vi "Filtering_and_Frequency_Domain.vi"() -> ()   [LabVIEW 2016]
uses:
  <vilib>/Analysis/2dsp.llb/Real FFT.vi
  <vilib>/Analysis/3filter.llb/Butterworth Filter (DBL).vi
  <vilib>/Analysis/NI_AALBase.lvlib
  <vilib>/Analysis/NI_AALPro.lvlib
panel:
  in  "Apply Filter?":bool=TRUE
  in  "Filter Type":T1(ring)
  in  "Low Cutoff Frequency (Hz)":i32=20
  in  "High Cutoff Frequency (Hz)":i32=45
  out "Frequency Domain Signal":cluster{i32, dbl, dbl[]}(graph)={0, 1.0, []}
  in  "Sample Rate (Hz)":dbl=200.0
  out "Time Domain Signal":cluster{i32, dbl, "sine wave":dbl[]}[](graph)
  in  "Frequency (Hz)":dbl=10.0
  in  "Signal Type":enum16{"Impulse", "Sine wave", "Square wave"}(ring)
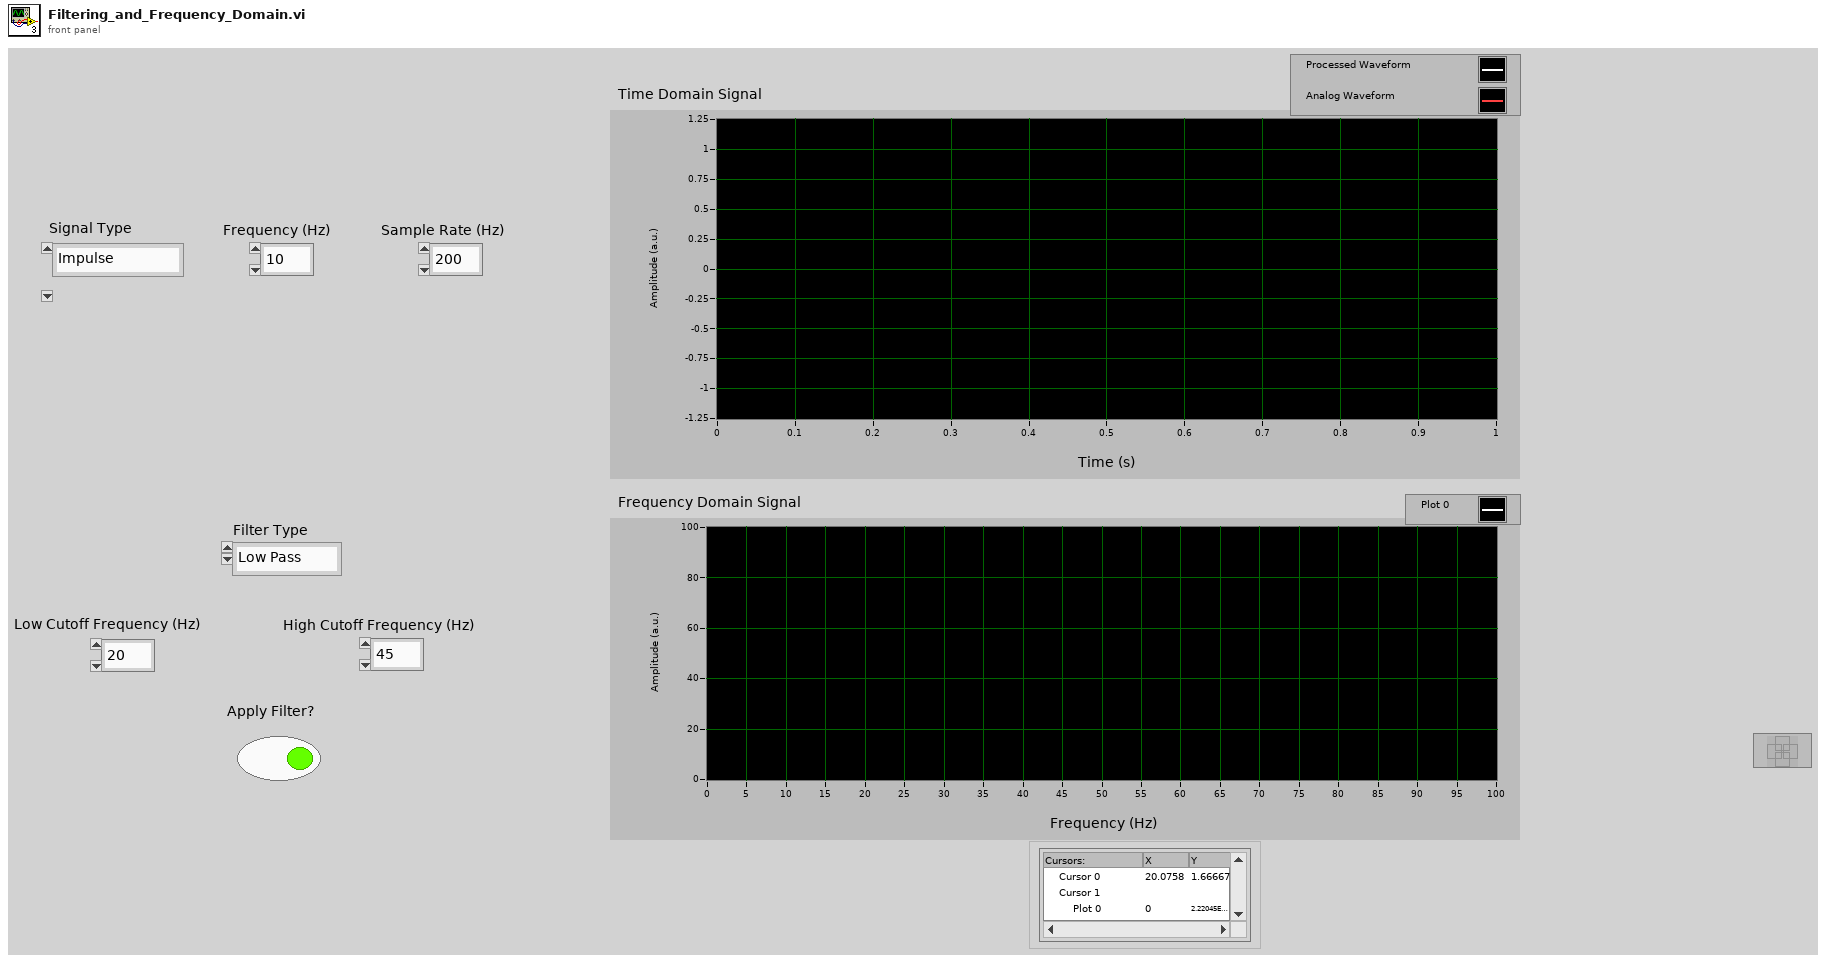
[diagram p1: front panel]
types:
  T1 = enum16{"Low Pass", "High Pass", "Band Pass", "Band Stop"}
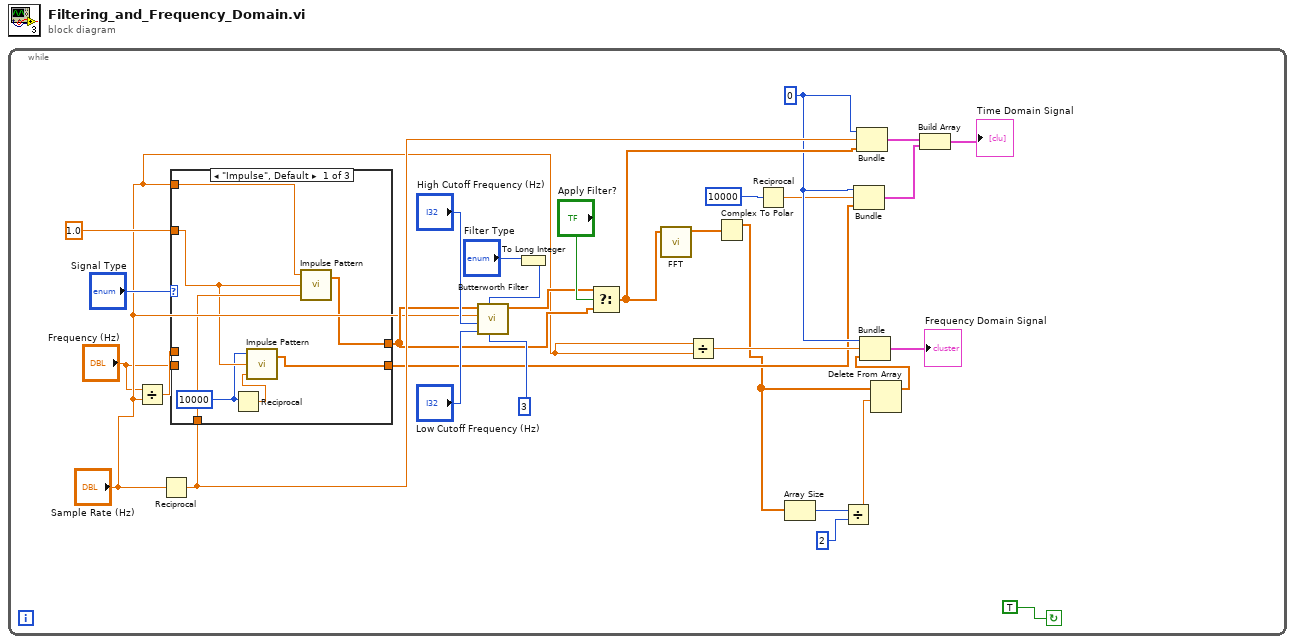
[diagram p0: block diagram]
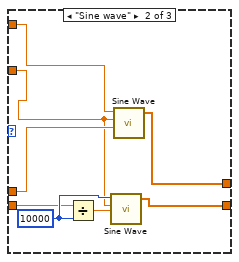
[diagram p2: hidden frame]
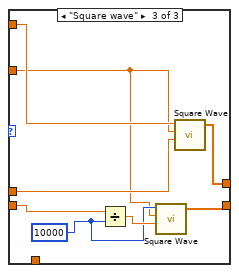
[diagram p3: hidden frame]
diagram:
  n1 = while {
    stop <- TRUE continue-if-true
    w9 = 0
    n2 = Divide(x="Frequency (Hz)", y="Sample Rate (Hz)") -> (x/y=w28:dbl)
    n3 = Reciprocal(x="Sample Rate (Hz)") -> (1/x=w24:dbl)
    n4 = case shown="\"Impulse\", Default" "Signal Type" {
      tunnel: "Sample Rate (Hz)" -> [w38 w42 w54]
      tunnel: 1.0 ("Signal Amplitude") -> [w35 w39 w49]
      tunnel: w28 -> [_ w45 w52]
      tunnel: [w36 w46 w53] -> w16
      tunnel: w24 -> [w37 _ _]
      tunnel: [w32 w41 w48] -> w8
      tunnel: "Frequency (Hz)" -> [_ w40 w47]
      frame "Impulse", Default {
        w33 = 10000
        n5 = Reciprocal(x=w33) -> (1/x=w34:dbl)
        n6 = call <vilib>:"Impulse Pattern.vi"("delay"=w34, "amplitude"=w35, "samples"=w33) -> ("Impulse Pattern"=w32:dbl[])  [unwired: 1 out]
        n7 = call <vilib>:"Impulse Pattern.vi"("delay"=w37, "amplitude"=w35, "samples"=w38) -> ("Impulse Pattern"=w36:dbl[])  [unwired: 1 out]
      }
      frame "Sine wave" {
        w43 = 10000
        n8 = Divide(x=w40, y=w43) -> (x/y=w44:dbl)
        n9 = call <vilib>:"Sine Wave.vi"("samples"=w43, "amplitude"=w39, "frequency"=w44) -> ("sine wave"=w41:dbl[])  [unwired: 2 in, 2 out]
        n10 = call <vilib>:"Sine Wave.vi"("samples"=w42, "amplitude"=w39, "frequency"=w45) -> ("sine wave"=w46:dbl[])  [unwired: 2 in, 2 out]
      }
      frame "Square wave" {
        w50 = 10000
        n11 = Divide(x=w47, y=w50) -> (x/y=w51:dbl)
        n12 = call <vilib>:"Square Wave.vi"("samples"=w50, "amplitude"=w49, "frequency"=w51) -> ("square wave"=w48:dbl[])  [unwired: 3 in, 2 out]
        n13 = call <vilib>:"Square Wave.vi"("samples"=w54, "amplitude"=w49, "frequency"=w52) -> ("square wave"=w53:dbl[])  [unwired: 3 in, 2 out]
      }
    }
    n14 = To Long Integer(number="Filter Type") -> (32bit integer=w19:i32)
    n15 = call-poly <vilib>:"Butterworth Filter.vi"("order"=3 ("Order"), "filter type"=w19, "low cutoff freq: fl"="Low Cutoff Frequency (Hz)", "high cutoff freq: fh"="High Cutoff Frequency (Hz)", "sampling freq: fs"="Sample Rate (Hz)", "X"=w16) -> ("Filtered X"=w17:dbl[])  [unwired: 1 in, 2 out]
    n16 = Select(t=w17, s="Apply Filter?", f=w16) -> (s? t:f=w11:dbl[])
    n17 = call-poly <vilib>:"FFT.vi"("X"=w11) -> ("FFT {X}"=w26:cdb[])  [unwired: 2 in, 8 out]
    n18 = Divide(x="Sample Rate (Hz)", y="Sample Rate (Hz)") -> (x/y=w27:dbl)
    n19 = Complex To Polar(r * e^(i*theta)=w26) -> (r=w1:dbl[])  [unwired: 1 out]
    n20 = Reciprocal(x=10000) -> (1/x=w4:dbl)
    n21 = Array Size(array=w1) -> (size(s)=w15:i32)
    n22 = Divide(x=w15, y=2) -> (x/y=w2:dbl)
    n23 = Bundle(w9, w4, "square wave"=w8) -> (w7:cluster{i32, dbl, "square wave":dbl[]})  [unwired: 1 out]
    n24 = Bundle(w9, w24, "square wave"=w11) -> (w10:cluster{i32, dbl, "square wave":dbl[]})  [unwired: 1 out]
    n25 = Delete From Array(array=w1, length=w2) -> (array with subset deleted=w13:dbl[])  [unwired: 1 in, 1 out]
    n26 = Bundle(w9, w27, w13) -> (→"Frequency Domain Signal":cluster{i32, dbl, dbl[]})  [unwired: 1 out]
    n27 = Build Array(w10, w7) -> (→"Time Domain Signal":cluster{i32, dbl, "square wave":dbl[]}[])
  }
